vi "FormAlarm.vi"() -> ()   [LabVIEW 2013]
panel:
  in  "枚举":enum16{"新消息", "已确认"}(ring)
  in  "删除":bool
  in  "确定":bool
  out "alarm":string[][](table)
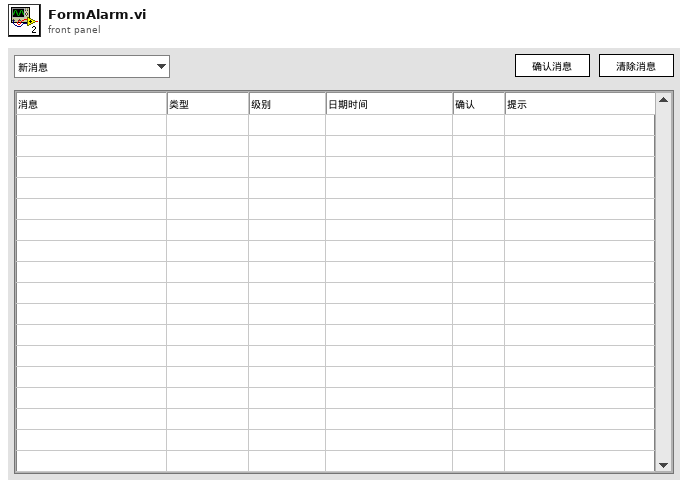
[diagram p1: front panel]
types:
  T1 = enum8{"Enabled", "Disabled", "Disabled and Grayed Out"}
  T2 = cluster{"userCode":string, "userName":string, "userStatus":string, "connectionMode":string}
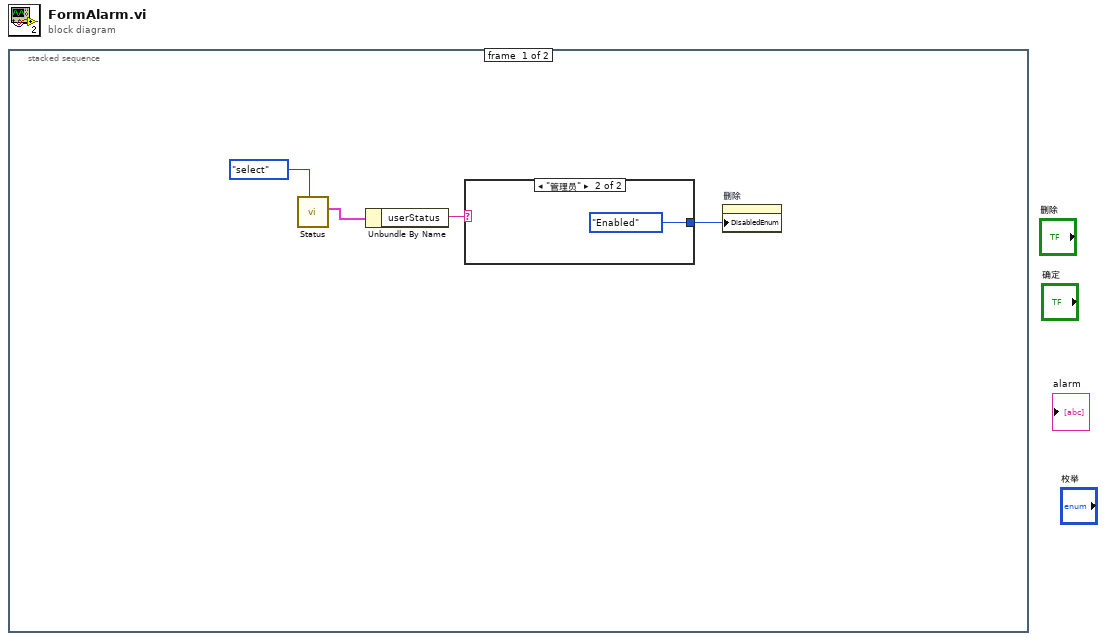
[diagram p0: block diagram]
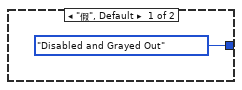
[diagram p2: hidden frame]
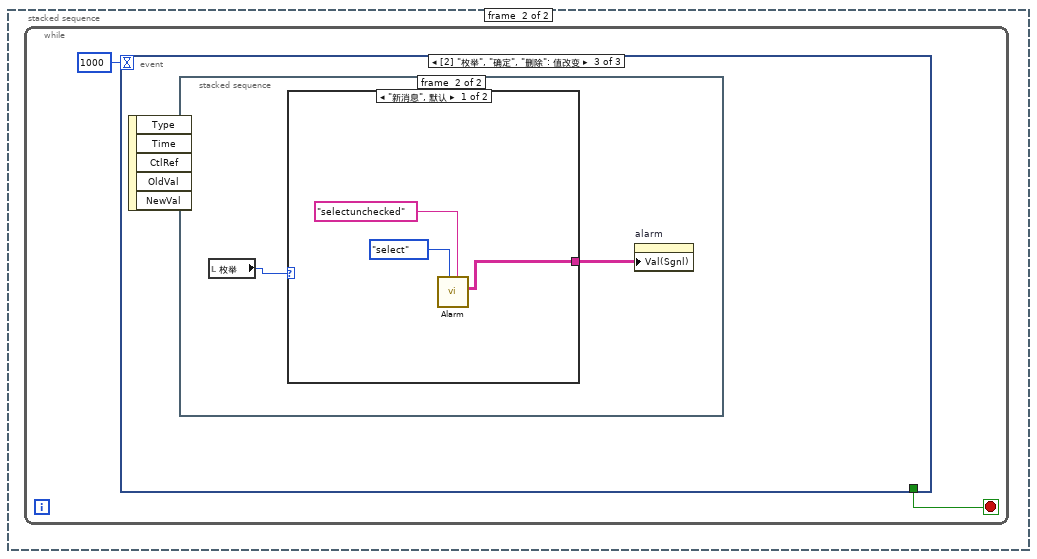
[diagram p3: hidden frame]
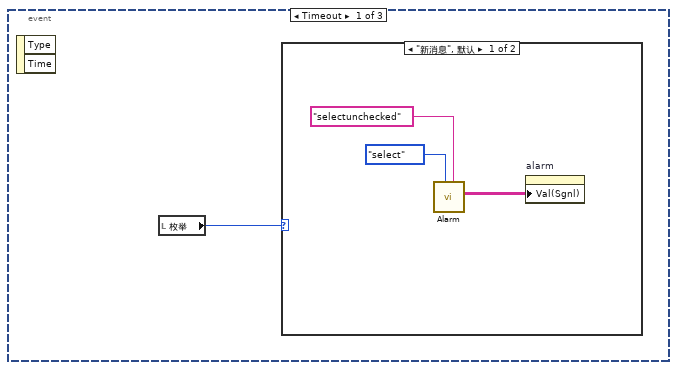
[diagram p4: hidden frame]
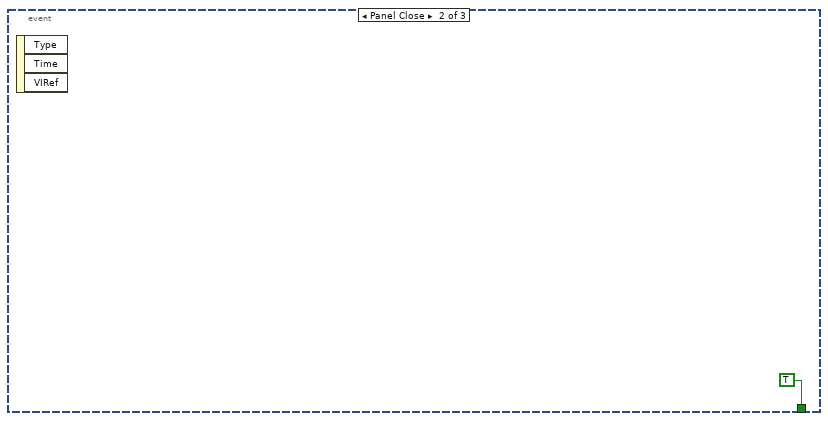
[diagram p6: hidden frame]
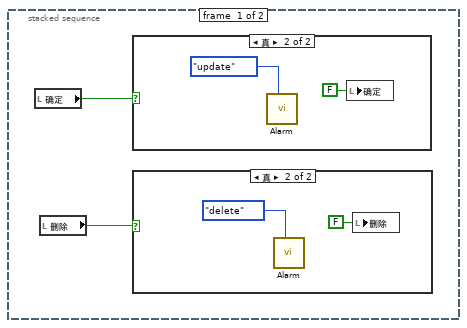
[diagram p7: hidden frame]
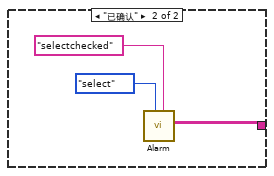
[diagram p10: hidden frame]
diagram:
  n1 = stacked-sequence {
    frame #0 {
      n2 = call "Status.vi"("模式"=enum16{"select", "insert", "update", "delete"}."select") -> ("元素"=w2:T2)  [unwired: 10 in]
      n3 = Unbundle By Name(w2) -> ("userStatus"=w4:string)
      n4 = case shown="\"管理员\"" w4 {
        tunnel: [T1."Disabled and Grayed Out" ("禁用") T1."Enabled" ("禁用")] -> w1
        frame "假", Default {
        }
        frame "管理员" {
        }
      }
      n5 = property on="删除" class="Bool (严格)"("DisabledEnum"=w1) -> ()  [unwired: 2 in, 2 out]
    }
    frame #1 {
      n6 = while {
        stop <- w8 stop-if-true
        n7 = event shown="[2] \"枚举\", \"确定\", \"删除\": 值改变" {
          selector: _ -> [_ _ _]
          dyn-events: _ -> [_ _ _]
          timeout: 1000 -> [_ _ _]
          tunnel: [_ TRUE _] -> w8
          event Timeout {
            n8 = event-data() -> ()  [unwired: 1 in, 2 out]
            n9 = local read "枚举"() -> (w9:enum16{"新消息", "已确认"})
            n10 = case shown="\"新消息\", 默认" w9 {
              frame "新消息", Default {
                n11 = call "Alarm.vi"("继承模式"="selectunchecked", "模式"=enum16{"select", "insert", "update", "delete"}."select") -> ("data"=w10:string[][])  [unwired: 9 in]
                n12 = property on="alarm" class="Tbl (严格)"("Val(Sgnl)"=w10) -> ()  [unwired: 2 in, 2 out]
              }
              frame "已确认" {
              }
            }
          }
          event Panel Close {
            n13 = event-data() -> ()  [unwired: 1 in, 3 out]
          }
          event "枚举", "确定", "删除": Value Change {
            n14 = event-data() -> ()  [unwired: 1 in, 5 out]
            n15 = stacked-sequence {
              frame #0 {
                n16 = local read "确定"() -> (w15:bool)
                n17 = local read "删除"() -> (w14:bool)
                n18 = case shown="真" w15 {
                  frame False {
                  }
                  frame True {
                    n19 = call "Alarm.vi"("模式"=enum16{"select", "insert", "update", "delete"}."update") -> ()  [unwired: 10 in, 1 out]
                    n20 = local write "确定"(FALSE ("确定")) -> ()
                  }
                }
                n21 = case shown="真" w14 {
                  frame False {
                  }
                  frame True {
                    n22 = call "Alarm.vi"("模式"=enum16{"select", "insert", "update", "delete"}."delete") -> ()  [unwired: 10 in, 1 out]
                    n23 = local write "删除"(FALSE ("删除")) -> ()
                  }
                }
              }
              frame #1 {
                n24 = local read "枚举"() -> (w20:enum16{"新消息", "已确认"})
                n25 = case shown="\"新消息\", 默认" w20 {
                  tunnel: [w22 w25] -> w21
                  frame "新消息", Default {
                    n26 = call "Alarm.vi"("继承模式"="selectunchecked", "模式"=enum16{"select", "insert", "update", "delete"}."select") -> ("data"=w22:string[][])  [unwired: 9 in]
                  }
                  frame "已确认" {
                    n27 = call "Alarm.vi"("继承模式"="selectchecked", "模式"=enum16{"select", "insert", "update", "delete"}."select") -> ("data"=w25:string[][])  [unwired: 9 in]
                  }
                }
                n28 = property on="alarm" class="Tbl (严格)"("Val(Sgnl)"=w21) -> ()  [unwired: 2 in, 2 out]
              }
            }
          }
        }
      }
    }
  }
